vi "Global Value RSim.vi"() -> ()   [LabVIEW 2017, in "NI_Robotics_Simulator.lvlib" / "NI_Robotics_Simulator Assistant.xnode"]
uses:
  <vilib>/robotics/Simulator/Interface/Simulator Xnode/NI_Robotics_Simulator Assistant.xnode
  <vilib>/robotics/Simulator/Interface/Simulator Xnode/SupportVIs/Controls/Assisant Configuration.ctl
panel:
  in  "CfgErrMsg_ReloadXMLFail":string="The following manifest file does not exist at the path you specified. \n%s\nYou must reconfigure and specify a valid path to a manifest file in the Simulator Assistant. "
  in  "Term_3DRefnum":string="3D picture refnum"
  in  "SAssErrMsg_OwnerNotSaved":string="Please save the main VI before you continue to use the Simulator Assistant."
  in  "SAssErrMsg_Multi-instances":string="If you have more than one <b>Simulation Assistant</b>, please keep only one instance."
  in  "SAssErrMsg_No_XML":string="The manifest file does not exist. It may have been moved or deleted. Please reconfigure the <b>Simulation Assistant</b> to specify the manifest file again."
  out "Assistant Configuration":T1
  in  "VI Name":string="Simulator Assistant"
  in  "Term_Done":string="done"
  in  "Term_Stop":string="stop"
  in  "Term_ErrOut":string="error out"
  in  "Term_ErrIn":string="error in (no error)"
  in  "CfgErrMsg_InvalidXMLFile":string="The manifest file for the simulation is empty or doesn't exist. Please select a valid xml file."
  in  "CfgErrMsg_InvalidStepSize":string="The step size for the simulation is invalid. The step size should be equal or greater than zero."
  in  "CfgErrMsg_UndefActuator":string="Please select model for the undefined actuator %s of robot %s. "
  in  "CfgErrMsg_UndefSensor":string="Please select model for the undefined sensor %s of robot %s. "
  in  "Undef Model":string="Undefined"
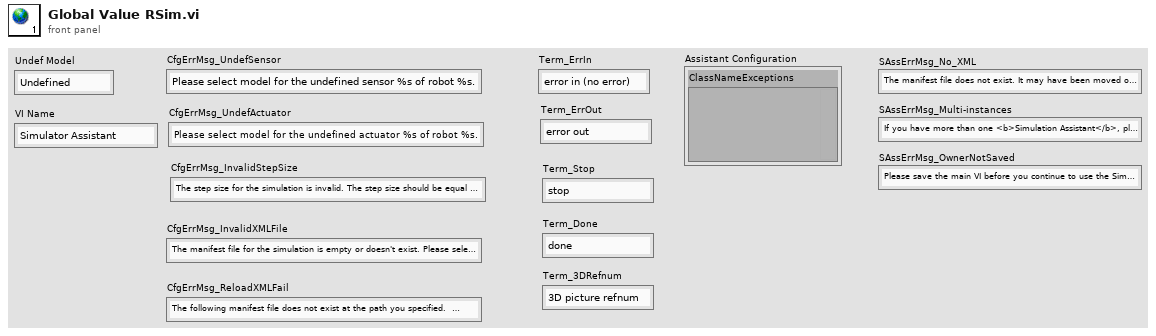
[diagram p1: front panel]
types:
  T1 = typedef "NI_Robotics_Simulator.lvlib/NI_Robotics_Simulator Assistant.xnode/Assisant Configuration.ctl" = cluster{"ClassNameExceptions":variant}
diagram:
